vi "Lab1_1.vi"() -> ()   [LabVIEW 2020]
panel:
  in  "Number of Points":dbl(knob)=8.0 min=8.0 max=1000.0 scale=8.0..1000.0
  out "Waveform Graph":dbl[](graph)
  out "Array":dbl[](array[numeric])
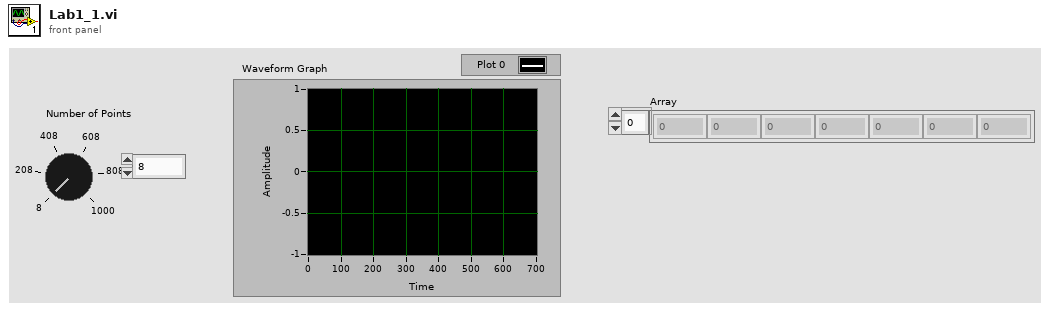
[diagram p1: front panel]
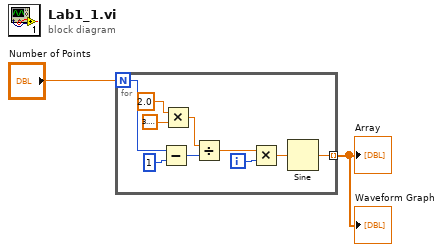
[diagram p0: block diagram]
diagram:
  n1 = for {
    N: "Number of Points" -> [w9]
    tunnel: [w12] -> w2 mode=indexing
    i -> [w6]
    n2 = Subtract(x=w9, y=1) -> (x-y=w8:i32)
    n3 = Multiply(x=2.0, y=3.141592653589793) -> (x*y=w5:dbl)
    n4 = Divide(x=w5, y=w8) -> (x/y=w11:dbl)
    n5 = Multiply(x=w11, y=w6) -> (x*y=w10:dbl)
    n6 = Sine(x=w10) -> (sin(x)=w12:dbl)
  }
  "Array" <- w2
  "Waveform Graph" <- w2
